vi "CCD Acquire Spectrum vs Wavenumbers.vi"(11 "error in":errorcluster) -> (15 "error out":errorcluster)   [LabVIEW 2020, in "Examples.lvlib"]
doc: "Example for a CCD spectrum acquisition."
uses:
  Examples.lvlib
  4aef6941-9f58-45d1-a797-2b486d7897ac.vi
  Classes/CCD/CCD.lvclass
  Classes/Mono/Monochromator.lvclass
  <vilib>/Utility/file.llb/Write Delimited Spreadsheet (DBL).vi
panel:
  out "XY Graph":cluster{"xAxis":dbl[], "imageData":dbl[]}(graph)
  # "Connector Pane"
  # "Locals"
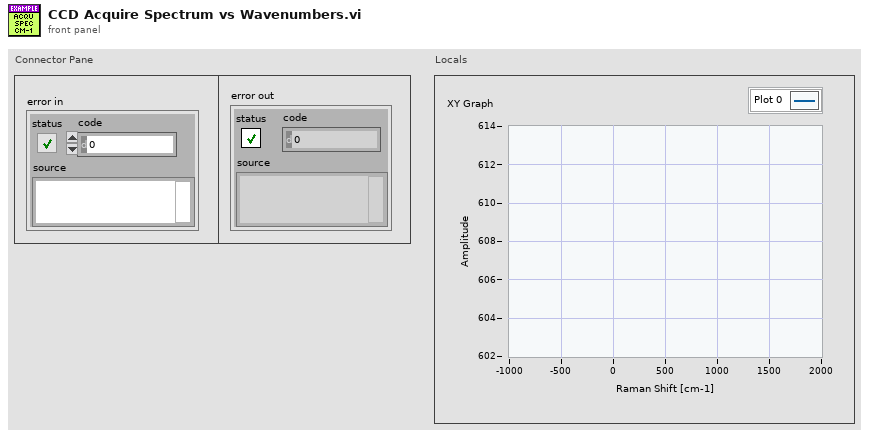
[diagram p1: front panel]
types:
  T1 = cluster{"ROI-index":i32, "xOrigin":i32, "yOrigin":i32, "xSize":i32, "ySize":i32, "xBin":i32, "yBin":i32}
  T2 = typedef "horiba.lvlib/CCD.lvclass/ccdAcquisitionData.ctl" = cluster{"acqIndex":i32, "ROIs":T3[], "timestamp":string}
  T3 = typedef "horiba.lvlib/CCD.lvclass/imageAcqData.ctl" = cluster{"roiMetaData":T4, "xAxis":dbl[], "yData":dbl[][]}
  T4 = typedef "horiba.lvlib/CCD.lvclass/roiMetaData.ctl" = cluster{"roiIndex":i32, "xBinning":i32, "xOrigin":i32, "xSize":i32, "yBinning":i32, "yOrigin":i32, "ySize":i32}
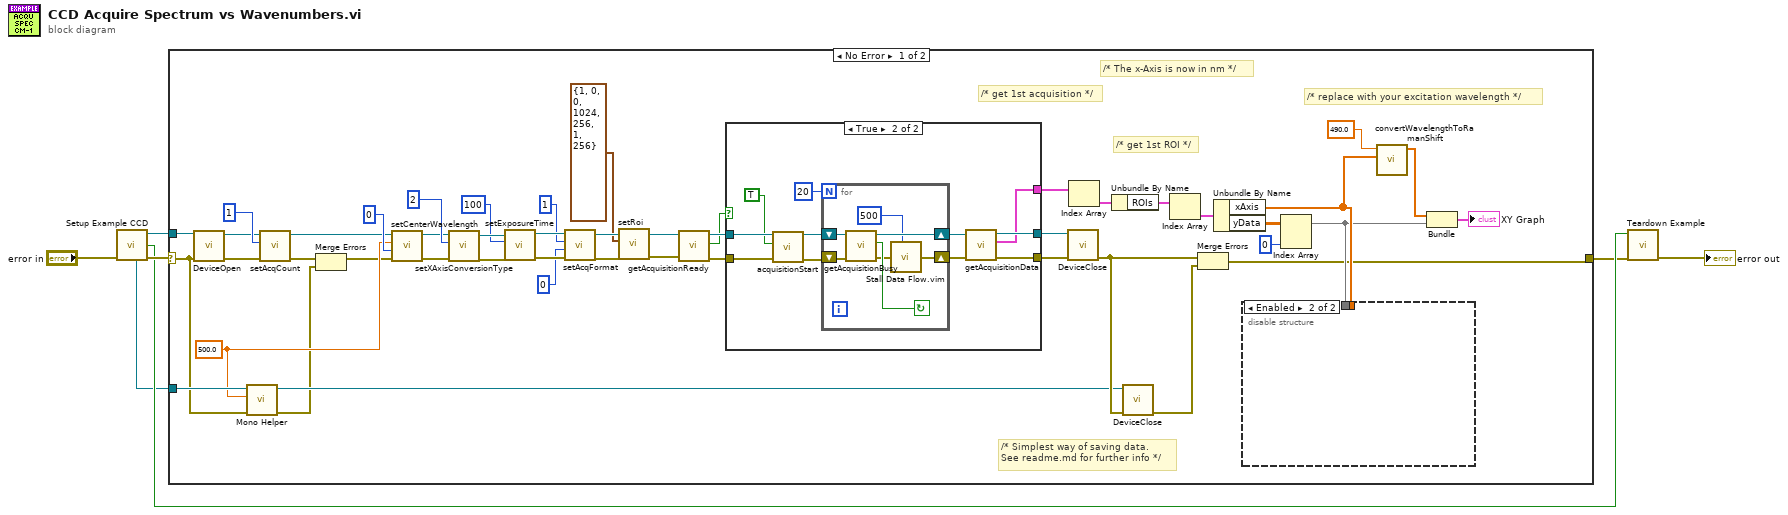
[diagram p0: block diagram]
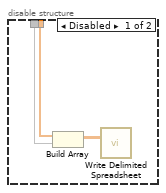
[diagram p2: hidden frame]
diagram:
  n1 = call "Setup Example CCD.vi"("error in (no error)"="error in") -> ("error out"=w5:errorcluster, "Module Was Already Running?"=w3:bool, "CCD out"=w4:refnum<class "CCD.lvclass">, "Mono out"=w1:refnum<class "Monochromator.lvclass">)  [unwired: 7 in]
  n2 = case shown="No Error" w5 {
    selector: w5 -> [w20 w78]
    tunnel: w4 -> [w30 _]
    tunnel: [w16 w78] -> w2
    tunnel: w1 -> [w21 _]
    frame No Error {
      w19 = 500.0 ("wavelength")
      # "/* replace with your excitation wavelength */"
      # "/* The x-Axis is now in nm */"
      # "/* Simplest way of saving data.\nSee readme.md for further info */"
      # "/* get 1st ROI */"
      # "/* get 1st acquisition */"
      n3 = call-dynamic "DeviceOpen.vi"("error in (no error)"=w20, "CCD in"=w30) -> ("error out"=w31:errorcluster, "CCD out"=w29:refnum<class "CCD.lvclass">)  [unwired: 6 in, 2 out]
      n4 = call "Mono Helper.vi"("error in (no error)"=w20, "wavelength in"=w19, "Monochromator in"=w21) -> ("error out"=w14:errorcluster, "Monochromator out"=w17:refnum<class "Monochromator.lvclass">)  [unwired: 6 in, 1 out]
      n5 = call "setAcqCount.vi"("error in (no error)"=w31, "count"=1, "CCD in"=w29) -> ("error out"=w53:errorcluster, "CCD out"=w10:refnum<class "CCD.lvclass">)  [unwired: 5 in, 2 out]
      n6 = Merge Errors(w53, w14) -> (w13:errorcluster)
      n7 = call "setCenterWavelength.vi"("error in (no error)"=w13, "monoIndex"=0, "wavelength"=w19, "CCD in"=w10) -> ("error out"=w12:errorcluster, "CCD out"=w11:refnum<class "CCD.lvclass">)  [unwired: 4 in, 2 out]
      n8 = call "setXAxisConversionType.vi"("error in (no error)"=w12, "type"=2, "CCD in"=w11) -> ("error out"=w51:errorcluster, "CCD out"=w50:refnum<class "CCD.lvclass">)  [unwired: 5 in, 2 out]
      n9 = call "setExposureTime.vi"("error in (no error)"=w51, "exposure time [ms] or [us]"=100, "CCD in"=w50) -> ("error out"=w48:errorcluster, "CCD out"=w47:refnum<class "CCD.lvclass">)  [unwired: 5 in, 2 out]
      n10 = call "setAcqFormat.vi"("error in (no error)"=w48, "format"=0, "number of ROIs"=1, "CCD in"=w47) -> ("error out"=w44:errorcluster, "CCD out"=w43:refnum<class "CCD.lvclass">)  [unwired: 4 in, 2 out]
      n11 = call "setRoi.vi"("error in (no error)"=w44, "roiConfig"=T1 {"ROI-index"=1, "xOrigin"=0, "yOrigin"=0, "xSize"=1024, "ySize"=256, "xBin"=1, "yBin"=256}, "CCD in"=w43) -> ("error out"=w9:errorcluster, "CCD out"=w8:refnum<class "CCD.lvclass">)  [unwired: 5 in, 2 out]
      n12 = call "getAcquisitionReady.vi"("error in (no error)"=w9, "CCD in"=w8) -> ("error out"=w42:errorcluster, "ready"=w40:bool, "CCD out"=w41:refnum<class "CCD.lvclass">)  [unwired: 7 in]
      n13 = case shown="True" w40 {
        tunnel: w42 -> [w58 w70]
        tunnel: w41 -> [w59 w69]
        tunnel: [w58 w63] -> w39
        tunnel: [w59 w61] -> w38
        tunnel: [_ w60] -> w36
        frame False {
        }
        frame True {
          n14 = call "acquisitionStart.vi"("error in (no error)"=w70, "openShutter"=TRUE, "CCD in"=w69) -> ("error out"=w65:errorcluster, "CCD out"=w64:refnum<class "CCD.lvclass">)  [unwired: 5 in, 2 out]
          n15 = for {
            N: 20 -> [_]
            shift-right: [w73] -> w66
            shift-left: w65 -> [w76]
            shift-right: [w72] -> w62
            shift-left: w64 -> [w77]
            stop <- w75 continue-if-true
            n16 = call "getAcquisitionBusy.vi"("error in (no error)"=w76, "CCD in"=w77) -> ("error out"=w74:errorcluster, "isBusy"=w75:bool, "CCD out"=w72:refnum<class "CCD.lvclass">)  [unwired: 7 in]
            n17 = call "Stall Data Flow.vim"("value in"=w74, "milliseconds to wait"=u32 500) -> ("value out"=w73:errorcluster)  [unwired: 1 out]
          }
          n18 = call "getAcquisitionData.vi"("error in (no error)"=w66, "CCD in"=w62) -> ("error out"=w63:errorcluster, "ccdAcquisitions"=w60:T2[], "CCD out"=w61:refnum<class "CCD.lvclass">)  [unwired: 6 in, 1 out]
        }
      }
      n19 = call-dynamic "DeviceClose.vi"("error in (no error)"=w39, "CCD in"=w38) -> ("error out"=w18:errorcluster)  [unwired: 5 in, 4 out]
      n20 = Index Array(array=w36) -> (element=w35:T2)  [unwired: 1 in]
      n21 = Unbundle By Name(w35) -> ("ROIs"=w34:T3[])
      n22 = call-dynamic "DeviceClose.vi"("error in (no error)"=w18, "Monochromator in"=w17) -> ("error out"=w15:errorcluster)  [unwired: 5 in, 4 out]
      n23 = Index Array(array=w34) -> (element=w33:T3)  [unwired: 1 in]
      n24 = Merge Errors(w18, w15) -> (w16:errorcluster)
      n25 = Unbundle By Name(w33) -> ("xAxis"=w25:dbl[], "yData"=w28:dbl[][])
      n26 = Index Array(array=w28, index (col)=0 ("disabled index (col)")) -> (element=w23:dbl[])  [unwired: 1 in]
      n27 = disable-structure shown="Enabled" {
        disable-tunnel: w25 -> [w57 _]
        disable-tunnel: w23 -> [w56 _]
        frame Disabled {
          n28 = Build Array(w57, w56) -> (w55:dbl[][])
          n29 = call-poly <vilib>:"Write Delimited Spreadsheet.vi"("2D data"=w55) -> ()  [unwired: 13 in, 2 out]
        }
        frame Enabled {
        }
      }
      n30 = call "convertWavelengthToRamanShift.vi"("wavelengths"=w25, "excitationWavelength"=490.0) -> ("Array"=w24:dbl[])  [unwired: 9 in]
      n31 = Bundle("Array"=w24, "yData"=w23) -> (→"XY Graph":cluster{"Array":dbl[], "yData":dbl[]})  [unwired: 1 in]
    }
    frame Error {
    }
  }
  n32 = call "Teardown Example.vi"("error in (no error)"=w2, "Module Was Already Running?"=w3) -> ("error out"=→"error out":errorcluster)  [unwired: 9 in]
